vi "Obtain Frame Buffer.vi"(7 "Buffer Size (10k)":i32=10000 format="%.0p", 8 "error in":errorcluster, 10 "Create (F)":bool) -> (0 "error out":errorcluster, 3 "queue out":refnum<queue>)   [LabVIEW 2025, in "Automotive Ethernet Bus Monitor.lvclass"]
doc: "Obtain the queue reference of the frame buffer queue."
uses:
  Automotive Ethernet Bus Monitor.lvclass
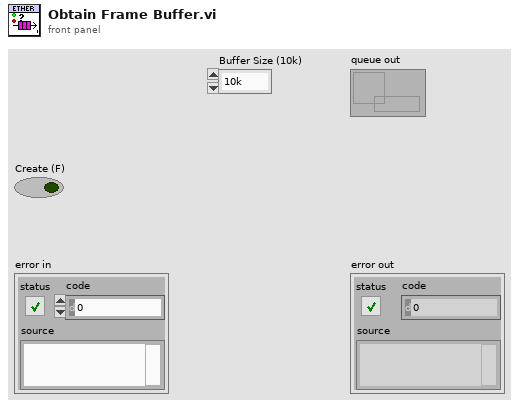
[diagram p1: front panel]
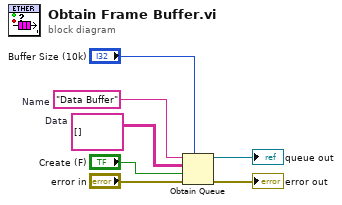
[diagram p0: block diagram]
diagram:
  w2 = string[][] []  # Data
  w3 = "Data Buffer"  # Name
  n1 = Obtain Queue(max queue size (-1, unlimited)="Buffer Size (10k)", name (unnamed)=w3, element data type=w2, create if not found? (T)="Create (F)", error in (no error)="error in") -> (queue out=→"queue out":refnum<queue>, error out=→"error out":errorcluster)  [unwired: 1 out]
